vi "KGN_Connect.vi"(7 "Serial Params in":T2={"Serial Settings:Baud Rate"=115200, "Serial Settings:Data Bits"=8, "Serial Settings:Parity"=0, "Serial Settings:Stop Bits"=10, "Serial Settings:Flow Control"=0, "Enable Termination Char (T)"=TRUE, "Message Based Settings:Termination Character"=3} {"Message Based Settings:Termination Character" format="%.0x"; "Serial Settings:Flow Control" items=["None", "XON/XOFF", "RTS/CTS", "XON/XOFF & RTS/CTS", "DTR/DSR", "XON/XOFF & DTR/DSR"]; "Serial Settings:Stop Bits" items=["1.0"=10, "1.5"=15, "2.0"=20]; "Serial Settings:Parity" items=["None", "Odd", "Even", "Mark", "Space"]}, 8 "Fehler (Eingang, kein Fehler)":errorcluster, 9 "Stopp":bool, 10 "serial port name":string="COM1", 11 "VISA-Ressourcenname":refnum<visa-resource-name>) -> (0 "Fehler (Ausgang)":errorcluster, 3 "VISA-Ressourcenname (Ausgang)":refnum<visa-resource-name>, 4 "Serial Params out":T1={"Serial Settings:Baud Rate"=0, "Serial Settings:Data Bits"=0, "Serial Settings:Parity"=0, "Serial Settings:Stop Bits"=10, "Serial Settings:Flow Control"=0, "Enable Termination Char (T)"=FALSE, "Message Based Settings:Termination Character"=0, "Serial Settings:End Mode for Reads"=0} {"Serial Settings:End Mode for Reads" items=["None", "Last Bit", "TermChar"]; "Serial Settings:Flow Control" items=["None", "XON/XOFF", "RTS/CTS", "XON/XOFF & RTS/CTS", "DTR/DSR", "XON/XOFF & DTR/DSR"]; "Serial Settings:Stop Bits" items=["1.0"=10, "1.5"=15, "2.0"=20]; "Serial Settings:Parity" items=["None", "Odd", "Even", "Mark", "Space"]}, 6 "Serial Params origin":T1={"Serial Settings:Baud Rate"=0, "Serial Settings:Data Bits"=0, "Serial Settings:Parity"=0, "Serial Settings:Stop Bits"=10, "Serial Settings:Flow Control"=0, "Enable Termination Char (T)"=FALSE, "Message Based Settings:Termination Character"=0, "Serial Settings:End Mode for Reads"=0} {"Serial Settings:End Mode for Reads" items=["None", "Last Bit", "TermChar"]; "Serial Settings:Flow Control" items=["None", "XON/XOFF", "RTS/CTS", "XON/XOFF & RTS/CTS", "DTR/DSR", "XON/XOFF & DTR/DSR"]; "Serial Settings:Stop Bits" items=["1.0"=10, "1.5"=15, "2.0"=20]; "Serial Settings:Parity" items=["None", "Odd", "Even", "Mark", "Space"]})   [LabVIEW 2020, in "Linearisierung v2.lvlib" / "Gasteiler.lvlib" / "HovaCAL_Interface.lvlib" / "KGN.lvlib"]
uses:
  KGN.lvlib
  Aktionen FGV Gasteiler Daten.ctl
  set/set.lvlib
  <vilib>/Instr/_visa.llb/VISA Configure Serial Port (Instr).vi
  Gasteiler.lvlib
  Helper/Helper.lvlib
panel:
  # "Endzeichen\n(0xA = '\\n' = LF)"
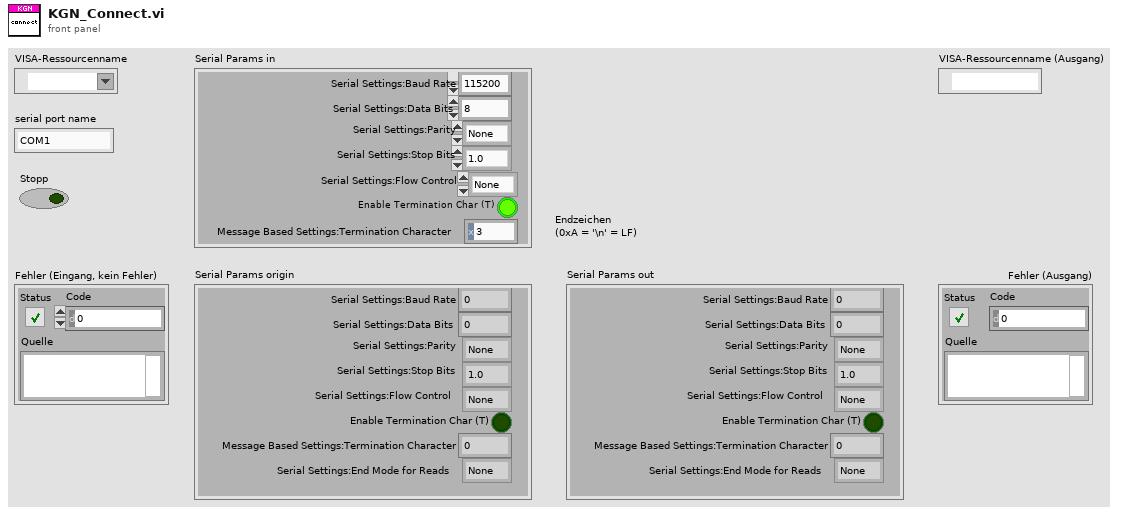
[diagram p1: front panel]
types:
  T1 = cluster{"Serial Settings:Baud Rate":u32, "Serial Settings:Data Bits":u16, "Serial Settings:Parity":u16, "Serial Settings:Stop Bits":u16, "Serial Settings:Flow Control":u16, "Enable Termination Char (T)":bool, "Message Based Settings:Termination Character":u8, "Serial Settings:End Mode for Reads":u16}
  T2 = cluster{"Serial Settings:Baud Rate":u32, "Serial Settings:Data Bits":u16, "Serial Settings:Parity":u16, "Serial Settings:Stop Bits":u16, "Serial Settings:Flow Control":u16, "Enable Termination Char (T)":bool, "Message Based Settings:Termination Character":u8}
  T3 = cluster{"Serial Settings:Baud Rate":u32, "Serial Settings:Data Bits":u16, "Serial Settings:Parity":u16, "Serial Settings:Stop Bits":u16, "Serial Settings:Flow Control":u16, "Message Based Settings:Termination Character Enable":bool, "Message Based Settings:Termination Character":u8, "Serial Settings:End Mode for Reads":u16}
  T4 = typedef "Linearisierung v2.lvlib/Gasteiler.lvlib/Aktionen FGV Gasteiler Daten.ctl" = enum16{"lesen", "Gasteiler Daten", "Seriellen Param.", "MB-Endwert", "laden", "speichern", "Anforderung", "TCP", "Aufzeichnung Start"}
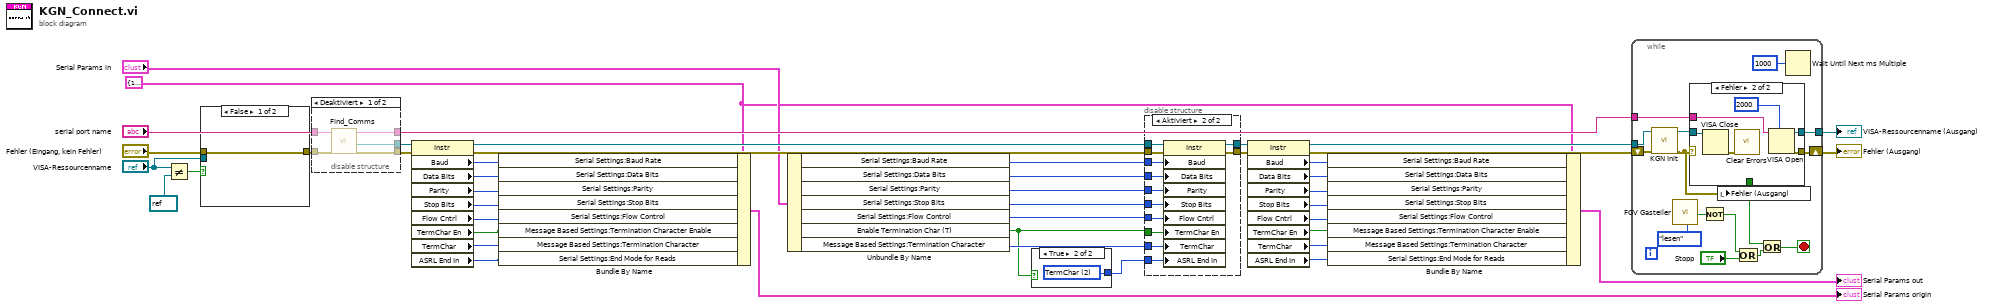
[diagram p0: block diagram]
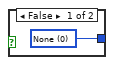
[diagram p2: hidden frame]
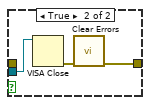
[diagram p3: hidden frame]
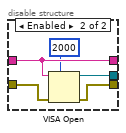
[diagram p4: hidden frame]
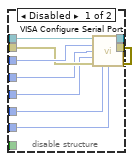
[diagram p5: hidden frame]
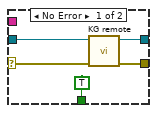
[diagram p6: hidden frame]
diagram:
  w1 = T3 {"Serial Settings:Baud Rate"=115200, "Serial Settings:Data Bits"=8, "Serial Settings:Parity"=0, "Serial Settings:Stop Bits"=10, "Serial Settings:Flow Control"=0, "Message Based Settings:Termination Character Enable"=FALSE, "Message Based Settings:Termination Character"=0, "Serial Settings:End Mode for Reads"=0} ("Serial Params in")
  n1 = Not Equal?(x="VISA-Ressourcenname", y=refnum<visa-resource-name> refnum ("VISA-Ressourcenname")) -> (x != y?=w17:bool)
  n2 = case shown="False" w17 {
    tunnel: "Fehler (Eingang, kein Fehler)" -> [w46 _]
    tunnel: [w46 w49] -> w18
    tunnel: "VISA-Ressourcenname" -> [_ w47]
    frame False {
    }
    frame True {
      n3 = VISA Close(VISA resource name=w47) -> (error out=w48:errorcluster)  [unwired: 1 in]
      n4 = call <vilib>:"Clear Errors.vi"("error in (no error)"=w48) -> ("error out"=w49:errorcluster)  [unwired: 5 in, 1 out]
    }
  }
  n5 = disable-structure shown="Deaktiviert" {
    disable-tunnel: [w54 w59] -> w43
    disable-tunnel: "serial port name" -> [w53 w56]
    disable-tunnel: w18 -> [w52 w58]
    disable-tunnel: [w51 w57] -> w28
    disable-tunnel: [w50 w56] -> w12
    frame Disabled {
      n6 = call "Find_Comms.vi"("Fehler (Eingang, kein Fehler)"=w52, "serial port name"=w53) -> ("Fehler (Ausgang)"=w51:errorcluster, "VISA-Referenz (Ausgang)"=w54:refnum<visa-resource-name>, "serial port name out"=w50:string)  [unwired: 6 in, 1 out]
    }
    frame Enabled {
      n7 = VISA Open(timeout (0)=u32 2000 ("VISA: Timeout bei Öffnen (0)"), error in (no error)=w58, VISA resource name=w56) -> (VISA resource name=w59:refnum<visa-resource-name>, error out=w57:errorcluster)  [unwired: 2 in]
    }
  }
  n8 = property class="Instr"(reference=w43, error in=w28) -> (reference out=w27:refnum<visa-resource-name>, error out=w26:errorcluster, "Baud"=w41:u32, "Data Bits"=w40:u16, "Parity"=w39:u16, "Stop Bits"=w38:u16, "Flow Cntrl"=w36:u16, "TermChar En"=w11:bool, "TermChar"=w5:u8, "ASRL End In"=w10:u16)
  n9 = Bundle By Name(cluster=w1, "Serial Settings:Baud Rate"=w41, "Serial Settings:Data Bits"=w40, "Serial Settings:Parity"=w39, "Serial Settings:Stop Bits"=w38, "Serial Settings:Flow Control"=w36, "Message Based Settings:Termination Character Enable"=w11, "Message Based Settings:Termination Character"=w5, "Serial Settings:End Mode for Reads"=w10) -> (→"Serial Params origin":T3)
  n10 = Unbundle By Name("Serial Params in") -> ("Serial Settings:Baud Rate"=w25:u32, "Serial Settings:Data Bits"=w24:u16, "Serial Settings:Parity"=w23:u16, "Serial Settings:Stop Bits"=w22:u16, "Serial Settings:Flow Control"=w21:u16, "Enable Termination Char (T)"=w3:bool, "Message Based Settings:Termination Character"=w9:u8)
  n11 = case shown="True" w3 {
    tunnel: [w60 w61] -> w2
    frame False {
      w60 = u16 0 items=["None", "Last Bit", "TermChar"] ("Serial Settings:End Mode for Reads")
    }
    frame True {
      w61 = u16 2 items=["None", "Last Bit", "TermChar"] ("Serial Settings:End Mode for Reads")
    }
  }
  n12 = disable-structure shown="Aktiviert" {
    disable-tunnel: [w70 w75] -> w30
    disable-tunnel: w27 -> [w68 w82]
    disable-tunnel: w26 -> [w66 w81]
    disable-tunnel: w25 -> [w67 w80]
    disable-tunnel: w24 -> [w65 w79]
    disable-tunnel: w23 -> [w64 w78]
    disable-tunnel: w22 -> [w63 w77]
    disable-tunnel: w21 -> [w62 w76]
    disable-tunnel: [w69 w74] -> w20
    disable-tunnel: w3 -> [_ w73]
    disable-tunnel: w9 -> [_ w72]
    disable-tunnel: w2 -> [_ w71]
    frame Disabled {
      n13 = call-poly "VISA Configure Serial Port"("VISA resource name"=w68, "baud rate (9600)"=w67, "data bits (8)"=w65, "parity (0:none)"=w64, "error in (no error)"=w66, "stop bits (10: 1 bit)"=w63, "flow control (0:none)"=w62) -> ("VISA resource name out"=w70:refnum<visa-resource-name>, "error out"=w69:errorcluster)  [unwired: 7 in]
    }
    frame Enabled {
      n14 = property class="Instr"(reference=w82, error in=w81, "Baud"=w80, "Data Bits"=w79, "Parity"=w78, "Stop Bits"=w77, "Flow Cntrl"=w76, "TermChar En"=w73, "TermChar"=w72, "ASRL End In"=w71) -> (reference out=w75:refnum<visa-resource-name>, error out=w74:errorcluster)
    }
  }
  n15 = property class="Instr"(reference=w30, error in=w20) -> (reference out=w13:refnum<visa-resource-name>, error out=w14:errorcluster, "Baud"=w35:u32, "Data Bits"=w34:u16, "Parity"=w33:u16, "Stop Bits"=w32:u16, "Flow Cntrl"=w31:u16, "TermChar En"=w8:bool, "TermChar"=w7:u8, "ASRL End In"=w6:u16)
  n16 = Bundle By Name(cluster=w1, "Serial Settings:Baud Rate"=w35, "Serial Settings:Data Bits"=w34, "Serial Settings:Parity"=w33, "Serial Settings:Stop Bits"=w32, "Serial Settings:Flow Control"=w31, "Message Based Settings:Termination Character Enable"=w8, "Message Based Settings:Termination Character"=w7, "Serial Settings:End Mode for Reads"=w6) -> (→"Serial Params out":T3)
  n17 = while {
    shift-right: [w95] -> w45
    shift-left: w14 -> [w92]
    tunnel: [w94] -> w44
    tunnel: w13 -> [w91]
    tunnel: w12 -> [w88]
    stop <- w96 stop-if-true
    n18 = call "KGN Init.vi"("Fehler (Eingang, kein Fehler)"=w92, "VISA-Ressourcenname"=w91) -> ("Fehler (Ausgang)"=w90:errorcluster, "VISA-Ressourcenname (Ausgang)"=w89:refnum<visa-resource-name>)  [unwired: 7 in, 1 out]
    n19 = call "FGV Gasteiler.vi"("Aktionen"=Aktionen_FGV_Gasteiler_Daten."lesen") -> ("Anforderung"=w84:bool)  [unwired: 11 in, 7 out]
    n20 = case shown="Fehler" w90 {
      selector: w90 -> [w98 _]
      tunnel: [TRUE _] -> w97
      tunnel: w89 -> [w101 w108]
      tunnel: [w99 w106] -> w95
      tunnel: [w100 w107] -> w94
      tunnel: w88 -> [_ w105]
      frame No Error {
        n21 = call "KG remote.vi"("Fehler (Eingang, kein Fehler)"=w98, "VISA-Ressourcenname"=w101) -> ("Fehler (Ausgang)"=w99:errorcluster, "VISA-Ressourcenname (Ausgang)"=w100:refnum<visa-resource-name>)  [unwired: 8 in]
      }
      frame Error {
        n22 = VISA Close(VISA resource name=w108) -> (error out=w104:errorcluster)  [unwired: 1 in]
        n23 = call <vilib>:"Clear Errors.vi"("error in (no error)"=w104) -> ()  [unwired: 5 in, 2 out]
        n24 = VISA Open(timeout (0)=u32 2000 ("VISA: Timeout bei Öffnen (0)"), VISA resource name=w105) -> (VISA resource name=w107:refnum<visa-resource-name>, error out=w106:errorcluster)  [unwired: 3 in]
      }
    }
    n25 = Not(x=w84) -> (.not. x?=w83:bool)
    n26 = local write "Fehler (Ausgang)"(w90) -> ()
    n27 = Or(x=w83, y="Stopp") -> (x .or. y?=w86:bool)
    n28 = Or(x=w97, y=w86) -> (x .or. y?=w96:bool)
    n29 = Wait Until Next ms Multiple(millisecond multiple=u32 1000 ("ms")) -> ()  [unwired: 1 out]
  }
  "Fehler (Ausgang)" <- w45
  "VISA-Ressourcenname (Ausgang)" <- w44
